vi "Write2Onenoe.vi"(1 "error in (no error)":errorcluster, 2 "strSendText":string) -> (0 "error out":errorcluster)   [LabVIEW 2014]
panel:
  in  "AutoItX3Lib.IAutoItX3":refnum<k7>
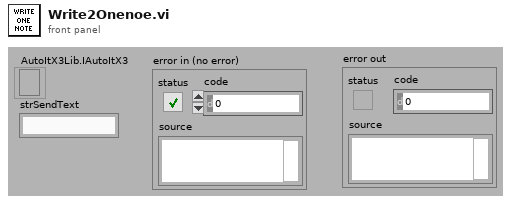
[diagram p1: front panel]
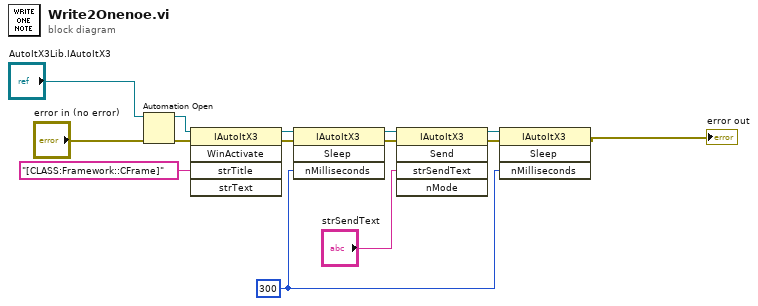
[diagram p0: block diagram]
diagram:
  w3 = 300 ("nTimeout")
  n1 = Automation Open(error in (no error)="error in (no error)", Automation Refnum="AutoItX3Lib.IAutoItX3") -> (Automation Refnum=w10:refnum<k7>, error out=w11:errorcluster)  [unwired: 2 in]
  n2 = invoke class="IAutoItX3" method="WinActivate"(reference=w10, error in=w11, "strTitle"="[CLASS:Framework::CFrame]") -> (reference out=w7:refnum<k7>, error out=w8:errorcluster)  [unwired: 2 in, 3 out]
  n3 = invoke class="IAutoItX3" method="Sleep"(reference=w7, error in=w8, "nMilliseconds"=w3) -> (reference out=w13:refnum<k7>, error out=w12:errorcluster)  [unwired: 1 in, 2 out]
  n4 = invoke class="IAutoItX3" method="Send"(reference=w13, error in=w12, "strSendText"="strSendText") -> (reference out=w5:refnum<k7>, error out=w4:errorcluster)  [unwired: 2 in, 3 out]
  n5 = invoke class="IAutoItX3" method="Sleep"(reference=w5, error in=w4, "nMilliseconds"=w3) -> (error out=→"error out":errorcluster)  [unwired: 1 in, 3 out]
